vi "Module - Template RT.vi"(8 "Error In":errorcluster) -> (0 "Error Out":errorcluster)   [LabVIEW 2020]
uses:
  Control/State - eFGV.ctl
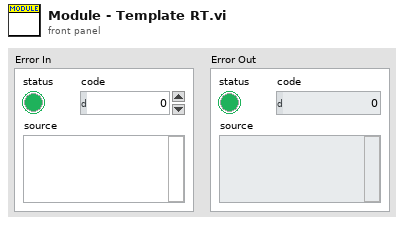
[diagram p1: front panel]
types:
  T1 = cluster{"T_Out":i32, "Event Ref":refnum<event-registration>}
  T2 = enum16{"Init", "Register Event", "Idle", "Process", "Close"}
  T3 = typedef "State - eFGV.ctl" = enum16{"Init", "Read", "Write", "Exit"}
  T4 = enum32{"invalid app kind", "Development System", "Run Time System", "Student Edition", "Embedded LabVIEW", "Evaluation", "Custom"}
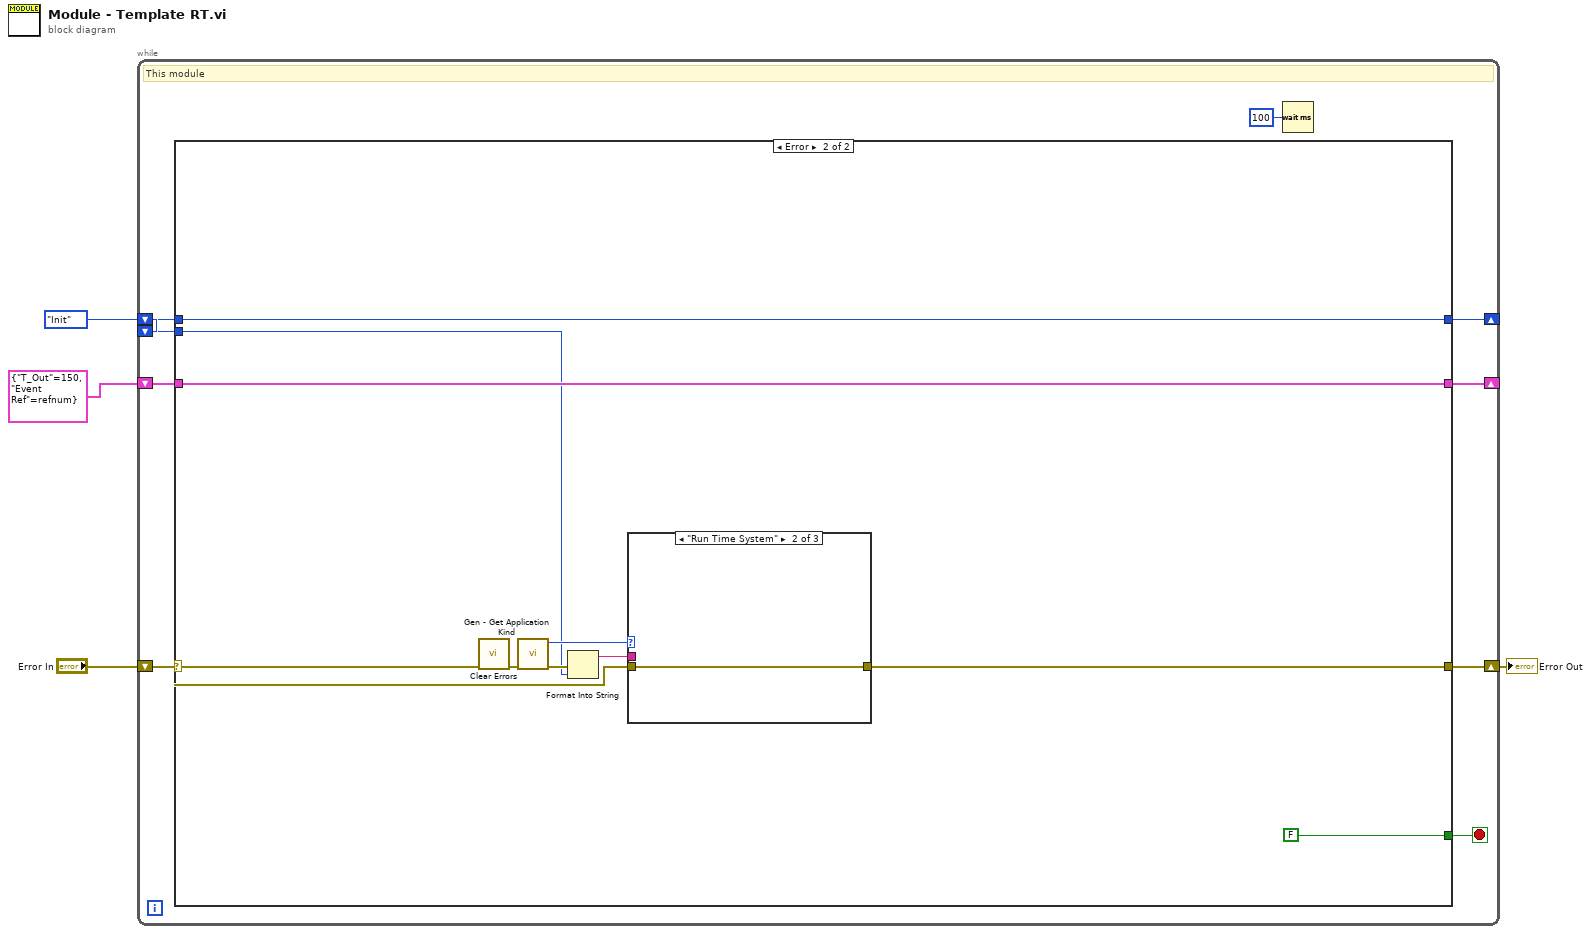
[diagram p0: block diagram]
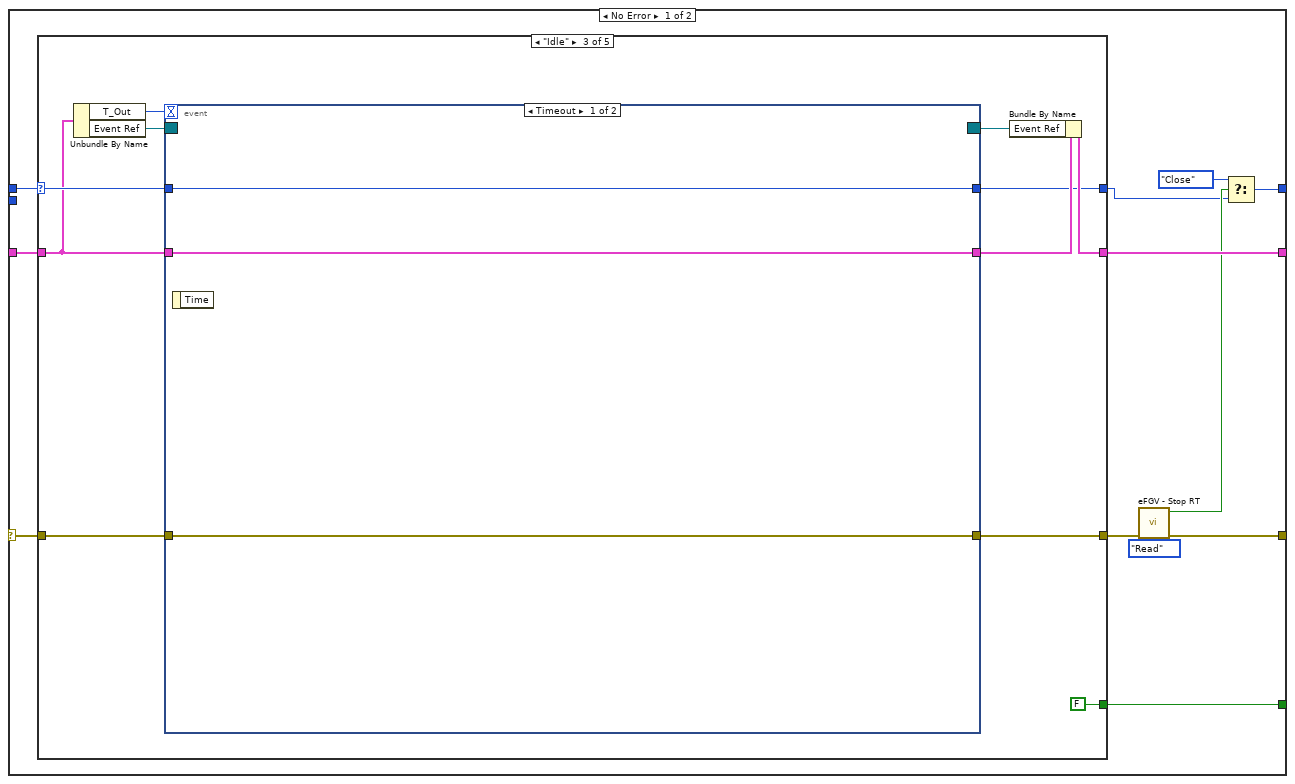
[diagram p2: hidden frame]
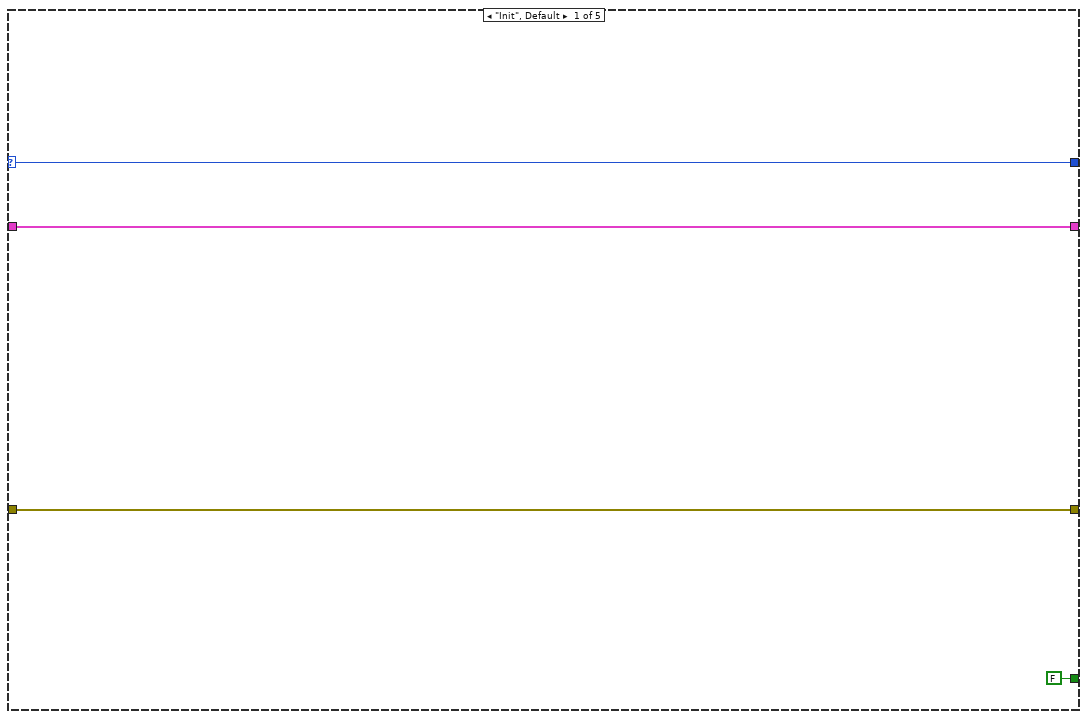
[diagram p3: hidden frame]
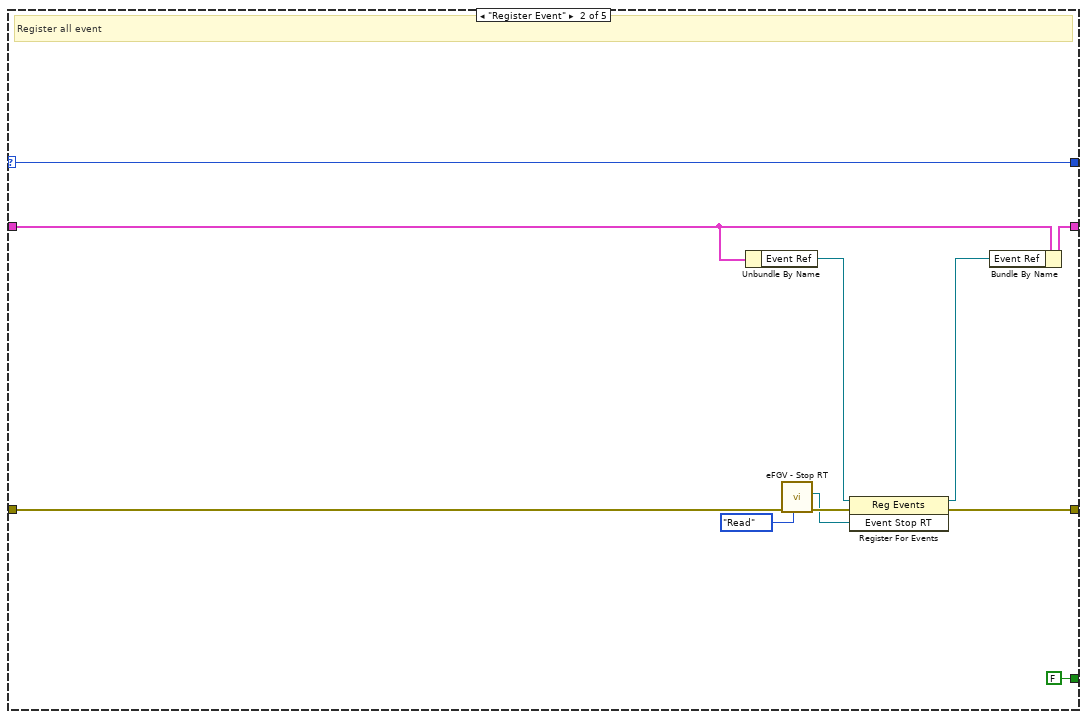
[diagram p4: hidden frame]
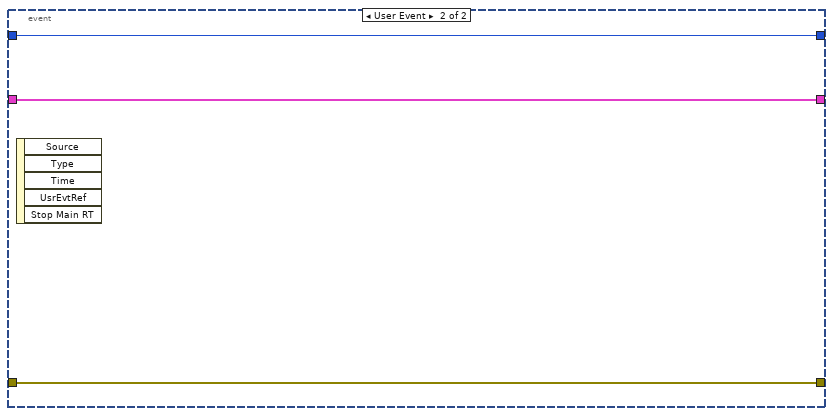
[diagram p5: hidden frame]
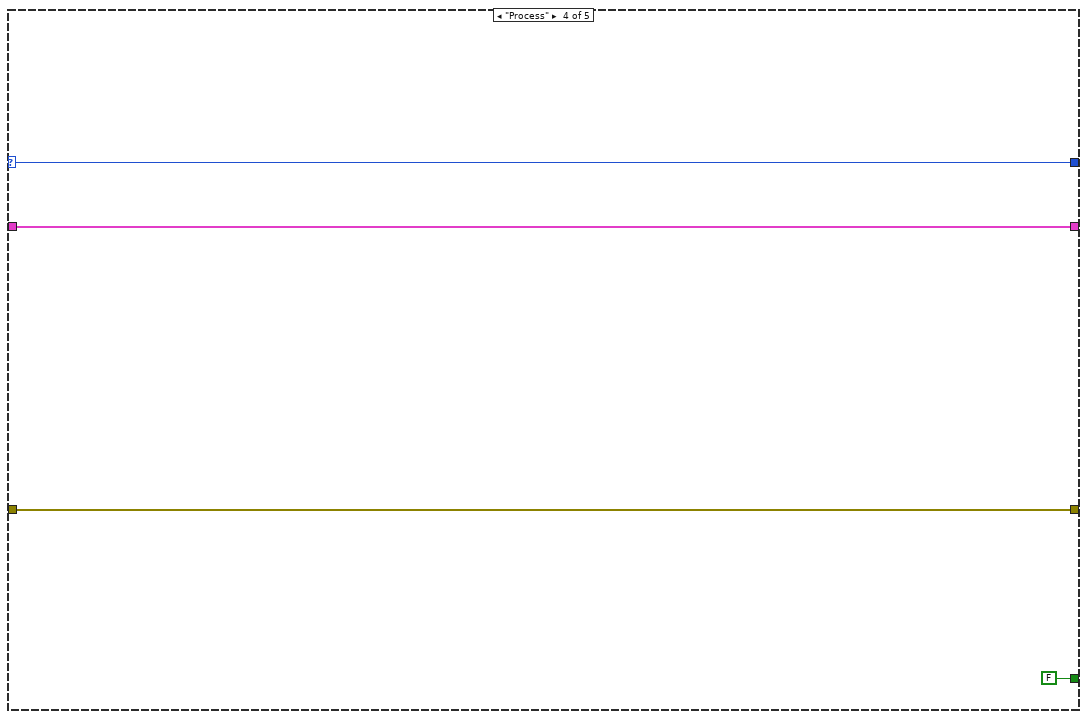
[diagram p6: hidden frame]
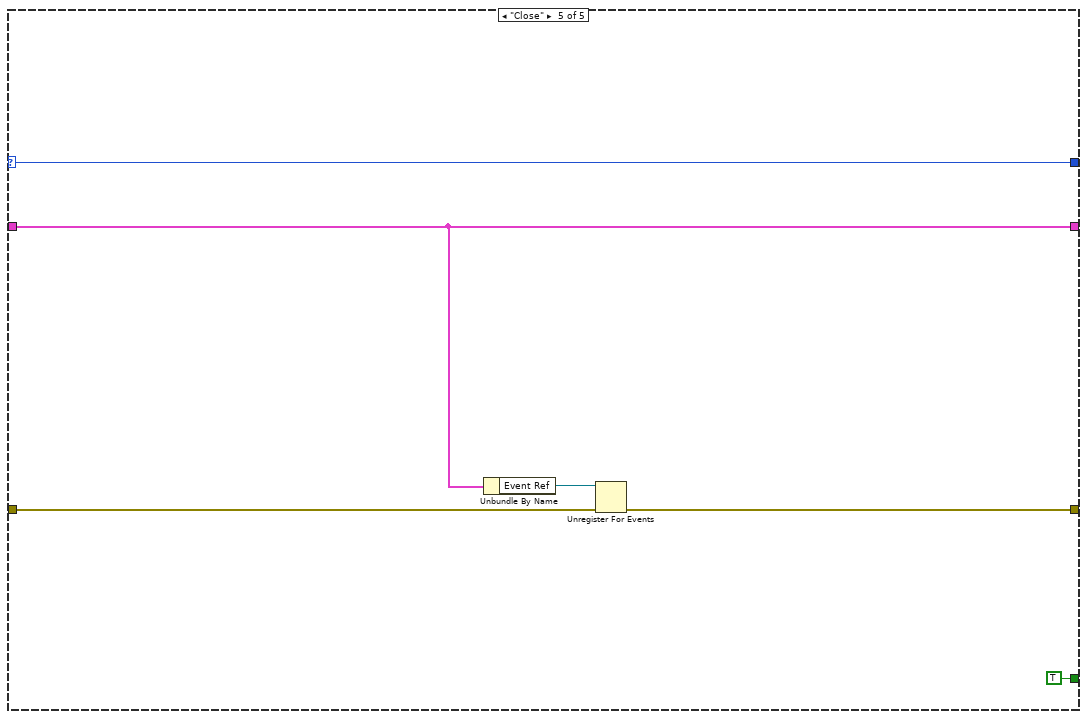
[diagram p7: hidden frame]
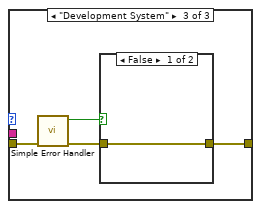
[diagram p9: hidden frame]
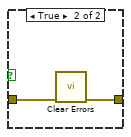
[diagram p10: hidden frame]
diagram:
  w1 = T2."Init"
  n1 = while {
    shift-right: [w9] -> _
    shift-left: w1 -> [w11]
    shift-right: [w12] -> w3
    shift-left: "Error In" -> [w13]
    shift-right: [w7] -> _
    shift-left: T1 {"T_Out"=150, "Event Ref"=refnum} -> [w8]
    shift-left: w1 -> [w5]
    stop <- w10 stop-if-true
    # "This module"
    n2 = case shown="Error" w13 {
      selector: w13 -> [w25 w75]
      tunnel: w11 -> [w24 w72]
      tunnel: [w19 w76] -> w12
      tunnel: [w23 FALSE] -> w10
      tunnel: [w14 w72] -> w9
      tunnel: w8 -> [w22 w71]
      tunnel: [w21 w71] -> w7
      tunnel: w5 -> [_ w69]
      frame No Error {
        n3 = case shown="\"Idle\"" w24 {
          selector: w24 -> [w26 w36 w47 w58 w65]
          tunnel: [w29 w40 w51 w61 w66] -> w20
          tunnel: w25 -> [w29 w38 w50 w61 w67]
          tunnel: [FALSE FALSE FALSE FALSE TRUE] -> w23
          tunnel: [w26 w36 w41 w58 w65] -> w15
          tunnel: w22 -> [w28 w34 w46 w59 w63]
          tunnel: [w28 w32 w43 w59 w63] -> w21
          frame "Init", Default {
          }
          frame "Register Event" {
            # "Register all event"
            n4 = Unbundle By Name(w34) -> ("Event Ref"=w33:refnum<event-registration>)
            n5 = call "eFGV - Stop RT.vi"("State"=State_-_eFGV."Read", "Error In"=w38) -> ("Error Out"=w39:errorcluster, "Event Stop RT"=w35:refnum<user-event>)  [unwired: 7 in, 1 out]
            n6 = register-events(reference=w33, error in=w39, w35) -> (reference out=w31:refnum<event-registration>, error out=w40:errorcluster)
            n7 = Bundle By Name(cluster=w34, "Event Ref"=w31) -> (w32:T1)
          }
          frame "Idle" {
            n8 = Unbundle By Name(w46) -> ("T_Out"=w45:i32, "Event Ref"=w44:refnum<event-registration>)
            n9 = event shown="[0] Timeout" {
              selector: w44 -> [_ _]
              dyn-events: [_ _] -> w42
              timeout: w45 -> [_ _]
              tunnel: [w54 w57] -> w51
              tunnel: w50 -> [w54 w57]
              tunnel: [w52 w55] -> w41
              tunnel: [w53 w56] -> w48
              tunnel: w46 -> [w53 w56]
              tunnel: w47 -> [w52 w55]
              event Timeout {
                n10 = event-data() -> ()  [unwired: 1 in, 1 out]
              }
              event User Event {
                n11 = event-data() -> ()  [unwired: 1 in, 5 out]
              }
            }
            n12 = Bundle By Name(cluster=w48, "Event Ref"=w42) -> (w43:T1)
          }
          frame "Process" {
          }
          frame "Close" {
            n13 = Unbundle By Name(w63) -> ("Event Ref"=w62:refnum<event-registration>)
            n14 = Unregister For Events(event registration refnum=w62, error in=w67) -> (error out=w66:errorcluster)
          }
        }
        n15 = call "eFGV - Stop RT.vi"("State"=State_-_eFGV."Read", "Error In"=w20) -> ("Error Out"=w19:errorcluster, "Stop RT? Out"=w17:bool)  [unwired: 7 in, 1 out]
        n16 = Select(t=T2."Close", s=w17, f=w15) -> (s? t:f=w14:T2)
      }
      frame Error {
        n17 = call <vilib>:"Clear Errors.vi"("error in (no error)"=w75) -> ("error out"=w77:errorcluster)  [unwired: 5 in, 1 out]
        n18 = call "Gen - Get Application Kind.vi"("Error In"=w77) -> ("Error Out"=w74:errorcluster, "Application:Kind"=w70:T4)  [unwired: 9 in]
        n19 = Format Into String(error in=w74, w69) -> (resulting string=w68:string)  [unwired: 2 in, 1 out]
        n20 = case shown="\"Run Time System\"" w70 {
          tunnel: [w78 w79 w83] -> w76
          tunnel: w75 -> [w78 w79 w81]
          tunnel: w68 -> [_ _ _]
          frame "invalid app kind", Default {
          }
          frame "Run Time System" {
          }
          frame "Development System" {
            n21 = call <vilib>:"Simple Error Handler.vi"("error in (no error)"=w81) -> ("error?"=w80:bool, "error out"=w82:errorcluster)  [unwired: 4 in, 3 out]
            n22 = case shown="False" w80 {
              tunnel: [w84 w86] -> w83
              tunnel: w82 -> [w84 w85]
              frame False {
              }
              frame True {
                n23 = call <vilib>:"Clear Errors.vi"("error in (no error)"=w85) -> ("error out"=w86:errorcluster)  [unwired: 5 in, 1 out]
              }
            }
          }
        }
      }
    }
    n24 = Wait (ms)(milliseconds to wait=u32 100) -> ()  [unwired: 1 out]
  }
  "Error Out" <- w3
